vi "Teleop.vi"(10 "Match Info":T1={"Autonomous Elapsed Seconds"=0.0, "TeleOp Elapsed Seconds"=0.0, "Disabled Elapsed Seconds"=0.0, "Visited Autonomous"=FALSE, "Visited TeleOp"=FALSE, "Visited Disabled"=FALSE, "Autonomous Settings"={"Autonomous Style"=enum."Independent", "VI Refnum"=refnum}}, 11 "Call Context":T2) -> ()   [LabVIEW 2018]
doc: "This VI is called for each enabled TeleOp packet received from the DS. It is typically used to read from joysticks and other inputs and update I/O or setpoints for timed control loops. It should complete and return within 20 milliseconds or risk missing DS packets."
uses:
  <vilib>/Rock Robotics/WPI/DriverStation/WPI_DriverStationDerivedRobotMode.ctl
  <vilib>/Rock Robotics/WPI/DriverStation/WPI_DriverStationMatch Info.ctl
  <vilib>/Rock Robotics/WPI/Solenoid/WPI_SolenoidValue.ctl
  Framework/Robot Global Data.vi
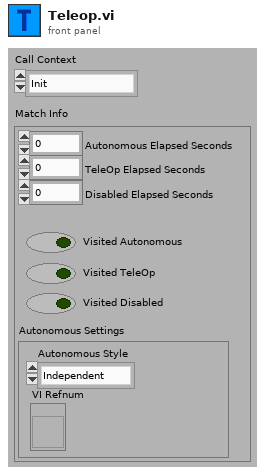
[diagram p1: front panel]
types:
  T1 = typedef "WPI_DriverStationMatch Info.ctl" = cluster{"Autonomous Elapsed Seconds":dbl, "TeleOp Elapsed Seconds":dbl, "Disabled Elapsed Seconds":dbl, "Visited Autonomous":bool, "Visited TeleOp":bool, "Visited Disabled":bool, "Autonomous Settings":cluster{"Autonomous Style":enum16{"Iterative", "Independent"}, "VI Refnum":refnum<vi>}}
  T2 = typedef "WPI_DriverStationDerivedRobotMode.ctl" = enum16{"Init", "Execute", "Stop"}
  T3 = typedef "Command Status Info.ctl" = cluster{"Name":string, "Status":T4, "notifier out":T5}
  T4 = typedef "Completion Status.ctl" = enum16{"Successful", "Aborted", "Incomplete"}
  T5 = typedef "Completion Notifier.ctl" = refnum<notifier>
  T6 = typedef "WPI_SolenoidValue.ctl" = enum16{"Off", "On", "Forward", "Reverse"}
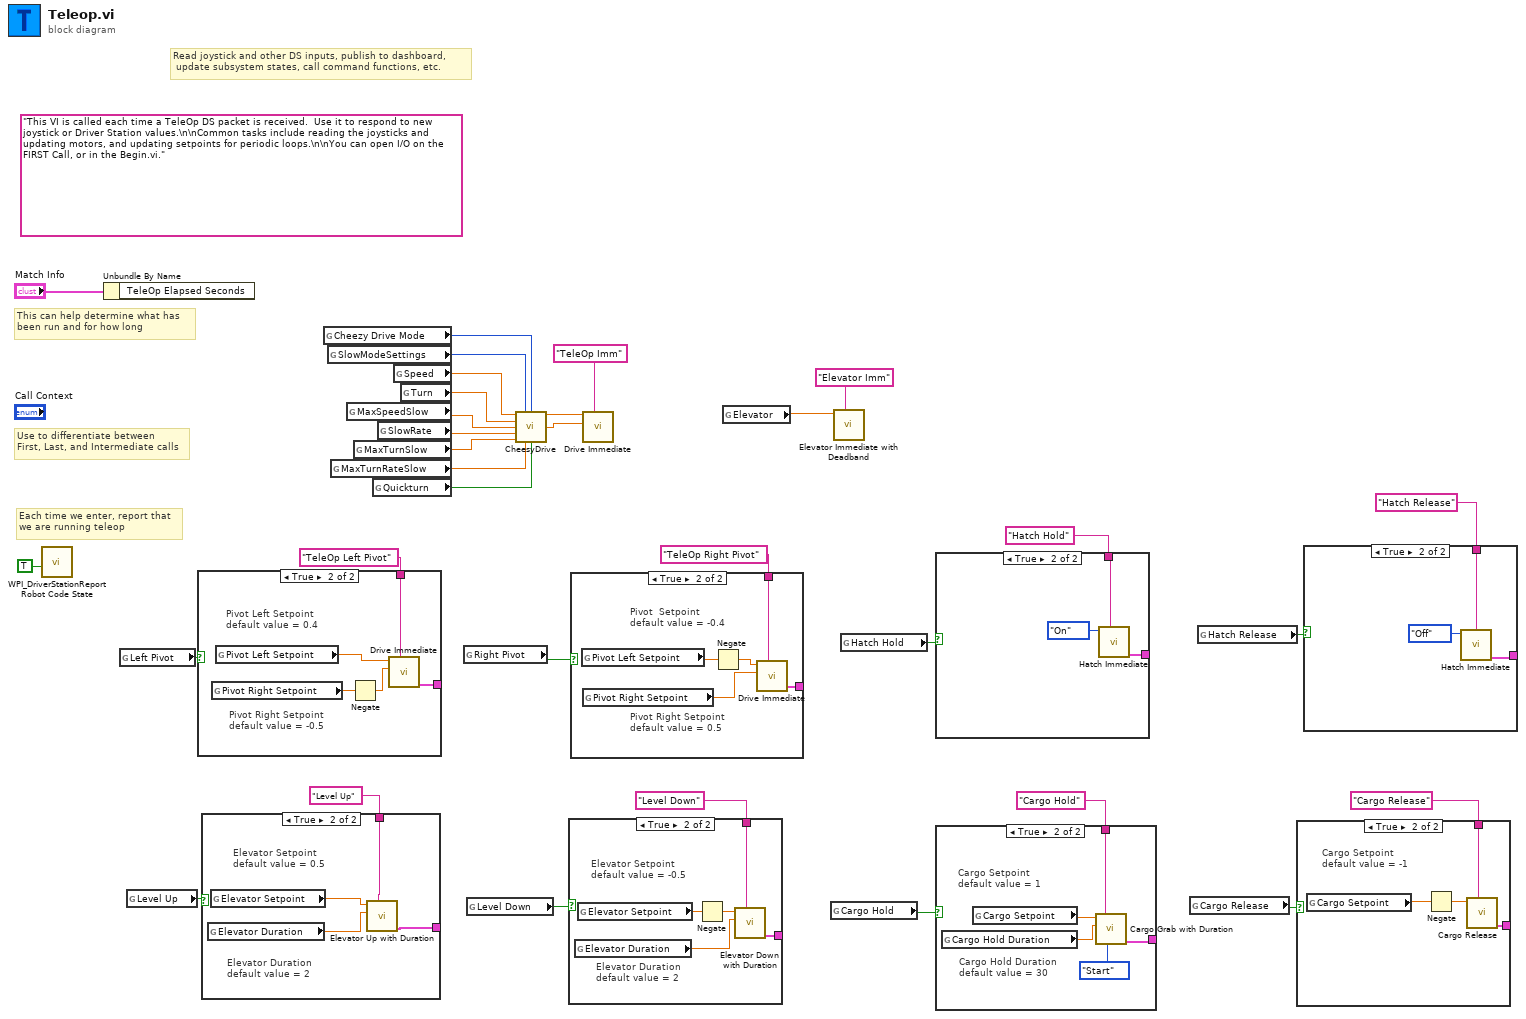
[diagram p0: block diagram]
diagram:
  (unwired) "This VI is called each time a TeleOp DS packet is received.  Use it to respond to new joystick or Driver Station values.\n\nCommon tasks include reading the joysticks and updating motors, and updating setpoints for periodic loops.\n\nYou can open I/O on the FIRST Call, or in the Begin.vi."
  # "Read joystick and other DS inputs, publish to dashboard,\n update subsystem states, call command functions, etc."
  # "Each time we enter, report that\nwe are running teleop"
  # "Use to differentiate between\nFirst, Last, and Intermediate calls"
  # "This can help determine what has\nbeen run and for how long"
  n1 = call <vilib>:"WPI_DriverStationReport Robot Code State.vi"("TeleOp"=TRUE ("Autonomous")) -> ()  [unwired: 10 in, 1 out]
  n2 = Unbundle By Name("Match Info") -> ()  [unwired: 1 out]
  n3 = global read "Robot Global Data.vi" "Left Pivot"() -> (w26:bool)
  n4 = global read "Robot Global Data.vi" "Level Up"() -> (w23:bool)
  n5 = case shown="True" w26 {
    tunnel: [_ w37] -> _
    tunnel: "TeleOp Left Pivot" ("Description") -> [_ w36]
    frame False {
    }
    frame True {
      # "Pivot Right Setpoint\ndefault value = -0.5"
      # "Pivot Left Setpoint\ndefault value = 0.4"
      n6 = global read "Robot Global Data.vi" "Pivot Right Setpoint"() -> (w34:dbl)
      n7 = global read "Robot Global Data.vi" "Pivot Left Setpoint"() -> (w35:dbl)
      n8 = Negate(x=w34) -> (-x=w33:dbl)
      n9 = call "Drive Immediate.vi"("Description"=w36, "Right Setpoint"=w33, "Left Setpoint"=w35) -> ("Command Info Out"=w37:T3)  [unwired: 8 in]
    }
  }
  n10 = case shown="True" w23 {
    tunnel: [_ w41] -> _
    tunnel: "Level Up" ("Description") -> [_ w40]
    frame False {
    }
    frame True {
      # "Elevator Setpoint\ndefault value = 0.5"
      # "Elevator Duration\ndefault value = 2"
      n11 = global read "Robot Global Data.vi" "Elevator Duration"() -> (w38:dbl)
      n12 = global read "Robot Global Data.vi" "Elevator Setpoint"() -> (w39:dbl)
      n13 = call "Elevator Up with Duration.vi"("Description"=w40, "Duration (s)"=w38, "Setpoint"=w39) -> ("Command Info Out"=w41:T3)  [unwired: 8 in]
    }
  }
  n14 = global read "Robot Global Data.vi" "Cheezy Drive Mode"() -> (w11:u32)
  n15 = global read "Robot Global Data.vi" "SlowModeSettings"() -> (w1:i32)
  n16 = global read "Robot Global Data.vi" "MaxTurnRateSlow"() -> (w3:dbl)
  n17 = global read "Robot Global Data.vi" "MaxSpeedSlow"() -> (w6:dbl)
  n18 = global read "Robot Global Data.vi" "MaxTurnSlow"() -> (w4:dbl)
  n19 = global read "Robot Global Data.vi" "Quickturn"() -> (w2:bool)
  n20 = global read "Robot Global Data.vi" "SlowRate"() -> (w5:dbl)
  n21 = global read "Robot Global Data.vi" "Speed"() -> (w8:dbl)
  n22 = global read "Robot Global Data.vi" "Turn"() -> (w7:dbl)
  n23 = global read "Robot Global Data.vi" "Right Pivot"() -> (w27:bool)
  n24 = global read "Robot Global Data.vi" "Level Down"() -> (w22:bool)
  n25 = call "CheesyDrive.vi"("Throttle"=w8, "SlowModeSettings"=w1, "SlowMode"=w11, "Wheel"=w7, "MaxSpeedSlow"=w6, "SlowRate"=w5, "MaxTurnSlow"=w4, "MaxTurnRateSlow"=w3, "Quickturn"=w2) -> ("Left PWM"=w10:dbl, "Right PWM"=w9:dbl)  [unwired: 5 in]
  n26 = case shown="True" w22 {
    tunnel: "Level Down" ("Description") -> [_ w46]
    tunnel: [_ w45] -> _
    frame False {
    }
    frame True {
      # "Elevator Duration\ndefault value = 2"
      # "Elevator Setpoint\ndefault value = -0.5"
      n27 = global read "Robot Global Data.vi" "Elevator Duration"() -> (w43:dbl)
      n28 = global read "Robot Global Data.vi" "Elevator Setpoint"() -> (w44:dbl)
      n29 = Negate(x=w44) -> (-x=w42:dbl)
      n30 = call "Elevator Down with Duration.vi"("Description"=w46, "Duration (s)"=w43, "Setpoint"=w42) -> ("Command Info Out"=w45:T3)  [unwired: 8 in]
    }
  }
  n31 = case shown="True" w27 {
    tunnel: [_ w51] -> _
    tunnel: "TeleOp Right Pivot" ("Description") -> [_ w50]
    frame False {
    }
    frame True {
      # "Pivot Right Setpoint\ndefault value = 0.5"
      # "Pivot  Setpoint\ndefault value = -0.4"
      n32 = global read "Robot Global Data.vi" "Pivot Left Setpoint"() -> (w48:dbl)
      n33 = global read "Robot Global Data.vi" "Pivot Right Setpoint"() -> (w49:dbl)
      n34 = Negate(x=w48) -> (-x=w47:dbl)
      n35 = call "Drive Immediate.vi"("Description"=w50, "Right Setpoint"=w49, "Left Setpoint"=w47) -> ("Command Info Out"=w51:T3)  [unwired: 8 in]
    }
  }
  n36 = call "Drive Immediate.vi"("Description"="TeleOp Imm", "Right Setpoint"=w9, "Left Setpoint"=w10) -> ()  [unwired: 8 in, 1 out]
  n37 = global read "Robot Global Data.vi" "Elevator"() -> (w17:dbl)
  n38 = global read "Robot Global Data.vi" "Cargo Hold"() -> (w19:bool)
  n39 = call "Elevator Immediate with Deadband.vi"("Description"="Elevator Imm", "Setpoint"=w17) -> ()  [unwired: 9 in, 1 out]
  n40 = global read "Robot Global Data.vi" "Hatch Hold"() -> (w12:bool)
  n41 = case shown="True" w12 {
    tunnel: "Hatch Hold" ("Description") -> [_ w54]
    tunnel: [_ w53] -> _
    frame False {
    }
    frame True {
      n42 = call "Hatch Immediate.vi"("Description"=w54, "Hatch Action"=WPI_SolenoidValue."On") -> ("Command Info Out"=w53:T3)  [unwired: 9 in]
    }
  }
  n43 = case shown="True" w19 {
    tunnel: [_ w59] -> _
    tunnel: "Cargo Hold" ("Description") -> [_ w58]
    frame False {
    }
    frame True {
      # "Cargo Hold Duration\ndefault value = 30"
      # "Cargo Setpoint\ndefault value = 1"
      n44 = global read "Robot Global Data.vi" "Cargo Hold Duration"() -> (w55:dbl)
      n45 = global read "Robot Global Data.vi" "Cargo Setpoint"() -> (w57:dbl)
      n46 = call "Cargo Grab with Duration.vi"("Synchronization"=enum16{"Start", "Wait"}."Start", "Description"=w58, "Duration (s)"=w55, "Setpoint"=w57) -> ("Command Info Out"=w59:T3)  [unwired: 7 in]
    }
  }
  n47 = global read "Robot Global Data.vi" "Cargo Release"() -> (w18:bool)
  n48 = global read "Robot Global Data.vi" "Hatch Release"() -> (w13:bool)
  n49 = case shown="True" w18 {
    tunnel: [_ w63] -> _
    tunnel: "Cargo Release" ("Description") -> [_ w62]
    frame False {
    }
    frame True {
      # "Cargo Setpoint\ndefault value = -1"
      n50 = global read "Robot Global Data.vi" "Cargo Setpoint"() -> (w61:dbl)
      n51 = Negate(x=w61) -> (-x=w60:dbl)
      n52 = call "Cargo Release.vi"("Description"=w62, "Setpoint"=w60) -> ("Command Info Out"=w63:T3)  [unwired: 9 in]
    }
  }
  n53 = case shown="True" w13 {
    tunnel: "Hatch Release" ("Description") -> [_ w66]
    tunnel: [_ w65] -> _
    frame False {
    }
    frame True {
      n54 = call "Hatch Immediate.vi"("Description"=w66, "Hatch Action"=WPI_SolenoidValue."Off") -> ("Command Info Out"=w65:T3)  [unwired: 9 in]
    }
  }
